vi "Inficon - Load recipe list.vi"(8 "Error In":errorcluster) -> (0 "Error Out":errorcluster, 2 "recipe list":string[](array[string]))   [LabVIEW 2014]
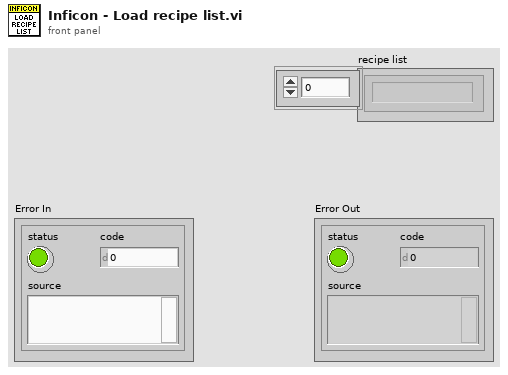
[diagram p1: front panel]
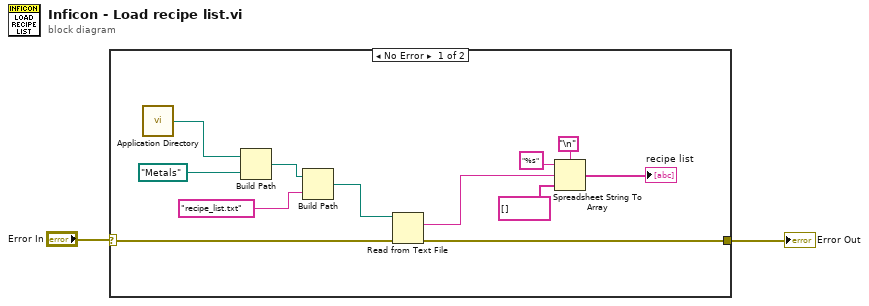
[diagram p0: block diagram]
diagram:
  n1 = case shown="No Error" "Error In" {
    selector: "Error In" -> [w4 w15]
    tunnel: [w3 w15] -> w1
    frame No Error {
      n2 = call <vilib>:"Application Directory.vi"() -> ("Application Directory"=w14:path)
      n3 = Build Path(base path=w14, name or relative path=path "Metals") -> (appended path=w13:path)
      n4 = Build Path(base path=w13, name or relative path="recipe_list.txt" ("string")) -> (appended path=w11:path)
      n5 = Read from Text File(file (use dialog)=w11, error in=w4) -> (text=w10:string, error out=w3:errorcluster)  [unwired: 2 in, 2 out]
      n6 = Spreadsheet String To Array(delimiter (Tab)="\n", format string="%s", spreadsheet string=w10, array type (2D Dbl)=string[] []) -> (array=→"recipe list":string[])
    }
    frame Error {
    }
  }
  "Error Out" <- w1
